vi "Configure Output Signal.vi"(8 "error in (no error)":errorcluster, 11 "Hardware Configuration In":T1={"Task ID"=0, "Volume"=0.0, "Sample Rate"=0.0, "Duration"=0, "Data"={"SignalType"=enum."SineWave", "Amplitude"=0.0, "WhiteNoiseSettings"={"Generate New Data"=FALSE, "Save"=FALSE, "Filter"=TRUE, "Gain"=0.0}, "SineWaveSttings"={"Frequency"=0.0}}, "Generated Data"={"t0"=timestamp(0 s since 1904-01-01), "dt"=1.0, "Y"=[]}} {"task ID out" format="%.0x"}) -> (0 "error out":errorcluster, 3 "Hardware Configuration Out":T1={"Task ID"=0, "Volume"=0.0, "Sample Rate"=0.0, "Duration"=0, "Data"={"SignalType"=enum."SineWave", "Amplitude"=0.0, "WhiteNoiseSettings"={"Generate New Data"=FALSE, "Save"=FALSE, "Filter"=TRUE, "Gain"=0.0}, "SineWaveSttings"={"Frequency"=0.0}}, "Generated Data"={"t0"=timestamp(0 s since 1904-01-01), "dt"=1.0, "Y"=[]}} {"task ID out" format="%.0x"})   [LabVIEW 2022 SP3]
doc: "Configure the hardware."
uses:
  Output Hardware Configuration.ctl
  <vilib>/sound2/lvsound2.llb/Sound Output Task ID.ctl
  Data.ctl
  WhiteNoiseSettings.ctl
  SineWaveSettings.ctl
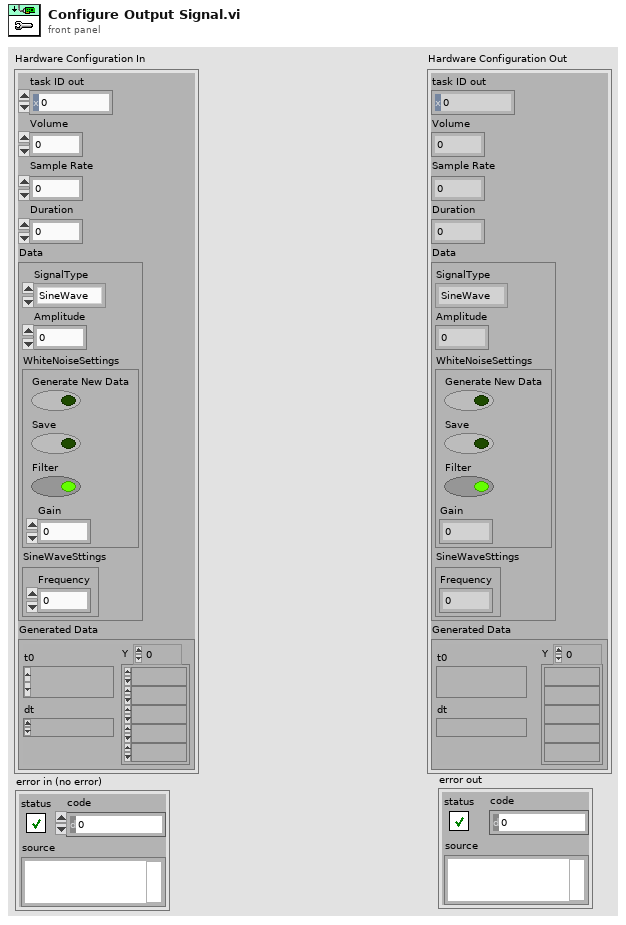
[diagram p1: front panel]
types:
  T1 = typedef "Output Hardware Configuration.ctl" = cluster{"Task ID":T2, "Volume":dbl, "Sample Rate":dbl, "Duration":i32, "Data":T3, "Generated Data":waveform(dbl)}
  T2 = typedef "Sound Output Task ID.ctl" = u32
  T3 = typedef "Data.ctl" = cluster{"SignalType":enum16{"WhiteNoise", "SineWave"}, "Amplitude":dbl, "WhiteNoiseSettings":T4, "SineWaveSttings":T5}
  T4 = typedef "WhiteNoiseSettings.ctl" = cluster{"Generate New Data":bool, "Save":bool, "Filter":bool, "Gain":dbl}
  T5 = typedef "SineWaveSettings.ctl" = cluster{"Frequency":dbl}
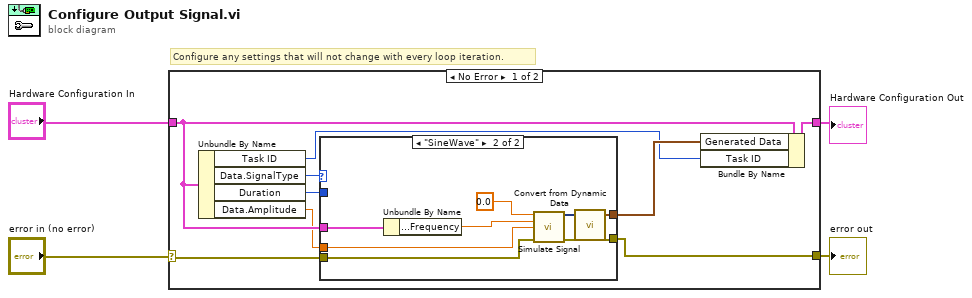
[diagram p0: block diagram]
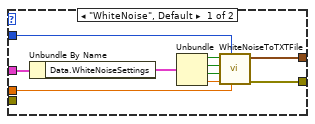
[diagram p2: hidden frame]
diagram:
  # "Configure any settings that will not change with every loop iteration."
  n1 = case shown="No Error" "error in (no error)" {
    selector: "error in (no error)" -> [w11 w33]
    tunnel: [w9 w33] -> w3
    tunnel: "Hardware Configuration In" -> [w13 w32]
    tunnel: [w10 w32] -> w1
    frame No Error {
      n2 = Unbundle By Name(w13) -> ("Task ID"=w7:T2, "Data.SignalType"=w12:enum16{"WhiteNoise", "SineWave"}, "Duration"=w6:i32, "Data.Amplitude"=w5:dbl)
      n3 = case shown="\"SineWave\"" w12 {
        tunnel: w13 -> [w23 w27]
        tunnel: [w17 w29] -> w9
        tunnel: [w16 w30] -> w8
        tunnel: w11 -> [_ w28]
        tunnel: w6 -> [w15 _]
        tunnel: w5 -> [w14 w24]
        frame "WhiteNoise", Default {
          n4 = Unbundle By Name(w23) -> ("Data.WhiteNoiseSettings"=w21:T4)
          n5 = Unbundle(w21) -> ("Generate New Data"=w22:bool, "Save"=w20:bool, "Filter"=w19:bool, "Gain"=w18:dbl)
          n6 = call "WhiteNoiseToTXTFile.vi"("standard deviation"=w14, "duration"=w15, "Gain"=w18, "Filter"=w19, "Save"=w20, "Generate New Data"=w22) -> ("error out"=w17:errorcluster, "output waveform"=w16:waveform(dbl))  [unwired: 4 in]
        }
        frame "SineWave" {
          n7 = Unbundle By Name(w27) -> ("Data.SineWaveSttings.Frequency"=w26:dbl)
          n8 = call "Simulate Signal"("Offset"=0.0, "Frequency"=w26, "Amplitude"=w24, "error in (no error)"=w28) -> ("Sine"=w31:dynamicdata, "error out"=w29:errorcluster)  [unwired: 10 in]
          n9 = call "Convert from Dynamic Data"("Dynamic Data Type"=w31) -> ("Waveform"=w30:waveform(dbl))  [unwired: 3 in]
        }
      }
      n10 = Bundle By Name(cluster=w13, "Generated Data"=w8, "Task ID"=w7) -> (w10:T1)
    }
    frame Error {
    }
  }
  "error out" <- w3
  "Hardware Configuration Out" <- w1
